vi "NACA_0015_Pressure_with_profile.vi"(3 "Mode":T5, 5 "Traverse line In":T1 {"Row Duration (mins)" format="%#.1f"; "Row No" min=0; "Trace Gas Concentration (%)" min=0.0 format="%#.2f"; "Emission Rate (l/min)" format="%#.2f"; "Tunnel Speed" format="%#.2f"; "Start X" format="%#.2f"; "Start Y" format="%#.2f"; "Start Z" format="%#.2f"; "End X" format="%#.2f"; "End Y" format="%#.2f"; "End Z" format="%#.2f"; "Averaging time (min)" min=0.0 format="%#.2f"}) -> (0 "Error Message":string, 1 "Status":T4, 2 "Traverse line Out":T1 {"Row Duration (mins)" format="%#.1f"; "Row No" min=0; "Trace Gas Concentration (%)" min=0.0 format="%#.2f"; "Emission Rate (l/min)" format="%#.2f"; "Tunnel Speed" format="%#.2f"; "Start X" format="%#.2f"; "Start Y" format="%#.2f"; "Start Z" format="%#.2f"; "End X" format="%#.2f"; "End Y" format="%#.2f"; "End Z" format="%#.2f"; "Averaging time (min)" min=0.0 format="%#.2f"})   [LabVIEW 2011]
uses:
  Gen Trav/Traverse_cluster.ctl
  Gen Trav/Spacing.ctl
  Controls/Multi_run_mode.ctl
  Controls/User_Specific_mode.ctl
  Gen Trav/Multi_Run_Status.ctl
  Gen Trav/Trav_mode.ctl
  Controls/Save_Data.ctl
  Controls/Setup.ctl
  <vilib>/Analysis/1siggen.llb/Ramp Pattern by Delta.vi
  <vilib>/Analysis/1siggen.llb/Ramp Pattern by Samples.vi
  Globals/Extra_Commands_Global.vi
  Globals/Meas_global.vi
  <vilib>/Analysis/NI_AALBase.lvlib
panel:
  out "Z":dbl
  out "Profile Points":cluster{dbl[], dbl[]}[](graph)
  out "Wake Profile":cluster{dbl[], dbl[]}(graph)
  in  "stop":bool
  out "Pressure":cluster{dbl[], dbl[]}(graph)
  out "Measurement No":i32
  # "X           Y            Z"
  # "Start"
  # "End"
  # "X           Y            Z"
  # "Start"
  # "End"
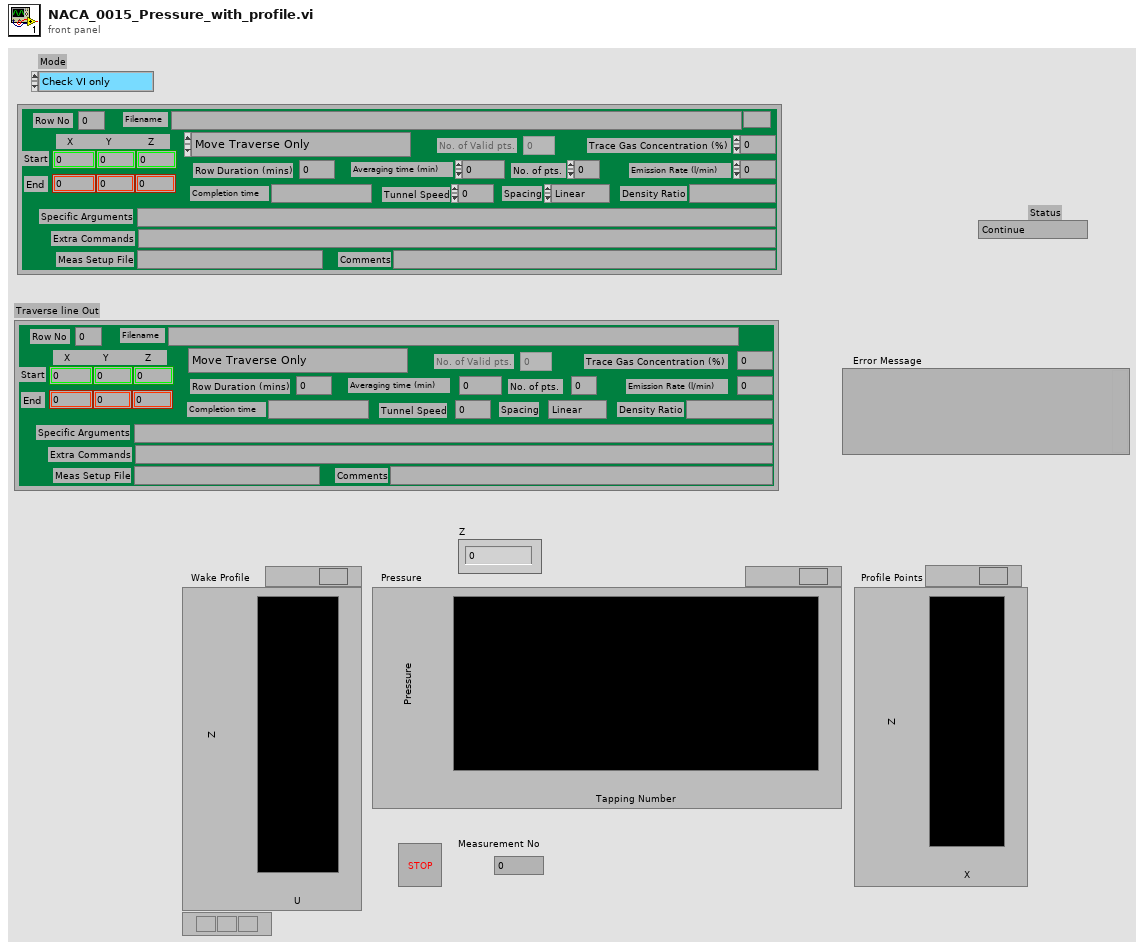
[diagram p1: front panel]
types:
  T1 = typedef "Traverse_cluster.ctl" = cluster{"Start X":dbl, "Start Y":dbl, "Start Z":dbl, "End X":dbl, "End Y":dbl, "End Z":dbl, "No. of pts.":i32, "Spacing":T2, "Filename":path, "Tunnel Speed":dbl, "Averaging time (min)":dbl, "Extra Commands":string, "Specific Arguments":string, "Emission Rate (l/min)":dbl, "Trace Gas Concentration (%)":dbl, "Density Ratio":string, "Comments":string, "Row No":i32, "Row Type Selector":T3, "Completion time":string, "Row Duration (mins)":dbl, "No. of Valid pts.":i32, "Meas Setup File":string}
  T2 = typedef "Spacing.ctl" = enum16{"Linear", "Log", "Gauss", "Specified", "N/A"}
  T3 = typedef "Multi_run_mode.ctl" = enum16{"Move Traverse Only", "Set Tunnel Speed Only", "Set Source Only", "Set Measurement Conditions", "Single Measurement", "Vertical Profile", "Lateral Profile", "Longitudinal Profile", "Explore Volume", "Multi-Axis Profile", "Auto Calibrate", "Meas Fast FID Bkgnd", "Check Beam Power", "Scanning Valve Measurement", "Run VI Named:", "Set ADAM Ch", "Wait (minutes)", "Send Message", "Synchronize With:", "Fall Back to this Row", "Turn Off Row Repeating", "Blank Row", "Traverse 3D Volume"}
  T4 = typedef "Multi_Run_Status.ctl" = enum16{"Continue", "Jump to Next Point", "Jump to Next Row", "Jump To Fall Back", "Terminate Run"}
  T5 = typedef "User_Specific_mode.ctl" = enum16{"Check VI only", "Run VI"}
  T6 = typedef "Trav_mode.ctl" = enum16{"Move traverse", "Read traverse position", "Teach Position"}
  T7 = typedef "Save_Data.ctl" = enum16{"Save No Data", "Save Data"}
  T8 = typedef "Setup.ctl" = enum16{"Run Program", "Show Setup", "Save Current Setup", "Setup Front Panel"}
  T9 = typedef "Status_Cluster.ctl" = cluster{"Status":T4, "Error Type":string, "Error Description":string}
  T10 = typedef "Analysis_info_cluster.ctl" = cluster{"Colour":u32, "Inst type":T11, "Inst name":string, "Symbol":string, "Code name":string, "Extra Info":string, "Inst Array":T12, "Extra Titles":string[], "Extra Values":string[], "U":dbl, "u^2":dbl, "u^3":dbl, "u^4":dbl, "Skew_u":dbl, "Kurt_u":dbl, "Sd Error in Mean":dbl, "% u'/U":dbl, "X":dbl, "Y":dbl, "Z":dbl, "Timescale integral to 25%":dbl, "Sd Error in Variance":dbl, "Calib File":path, "Calib Constants":dbl[], "Output Position":bool, "Full Stats":bool, "Av Sampling Rate":dbl, "Av No of Samples":dbl, "Total Meas Time (s)":dbl, "ADAM Ch Name":string}
  T11 = typedef "Inst_type.ctl" = enum16{"Propeller anemometer", "Raw voltage", "Pressure Transducer", "Pitot-static tube", "Preston tube", "Hot wire", "Cross wire 1", "Cross wire 2", "Generic Linear", "Generic Polynomial", "Generic BackPoly", "Fast FID", "Thermocouple", "Cold wire", "Pulsed Wire", "LDA Vel", "LDA Tran time", "LDA Arr time"}
  T12 = typedef "Instrument_Array.ctl" = enum16{"PWA", "LDA", "Analogue"}
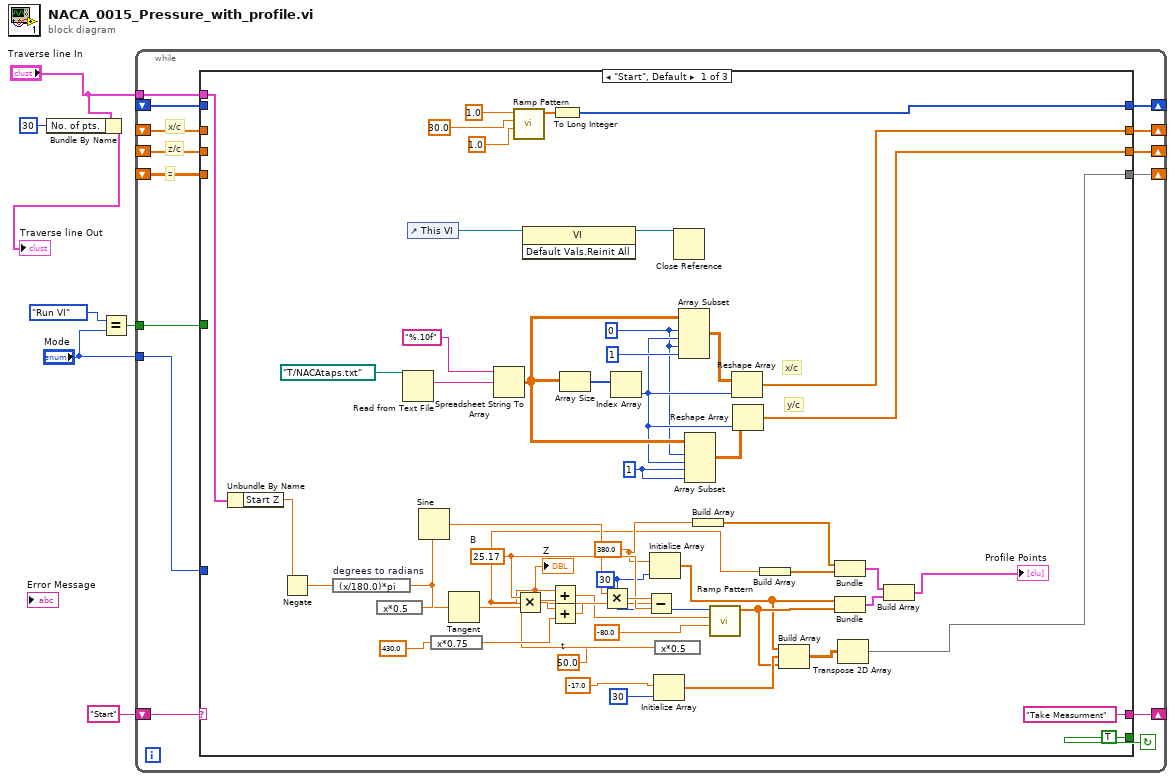
[diagram p0: block diagram]
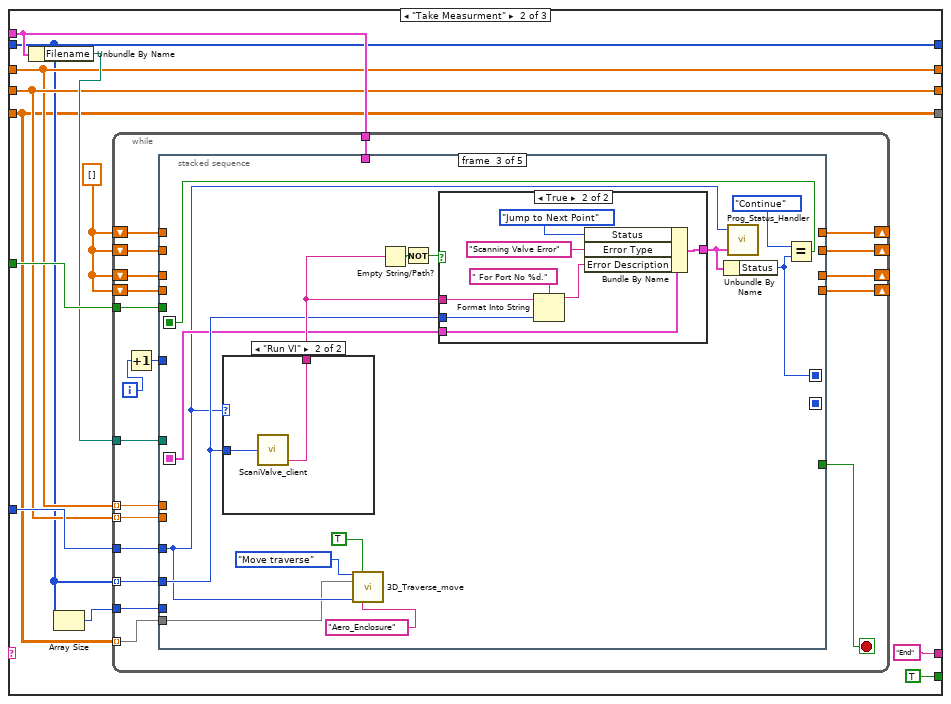
[diagram p2: hidden frame]
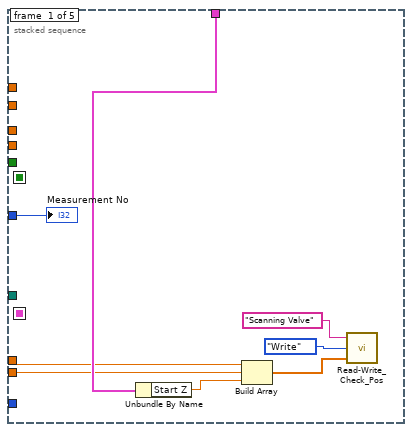
[diagram p3: hidden frame]
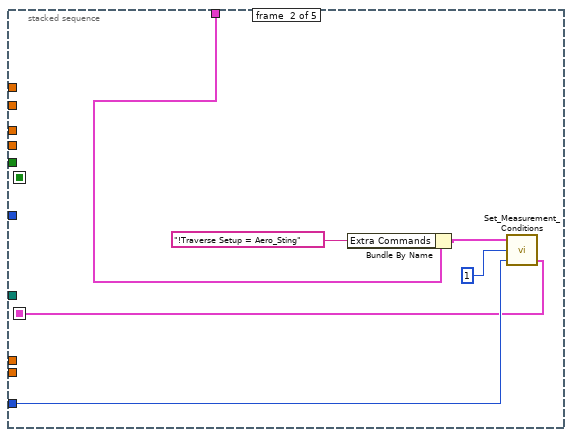
[diagram p4: hidden frame]
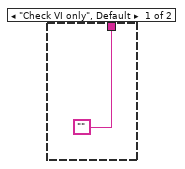
[diagram p5: hidden frame]
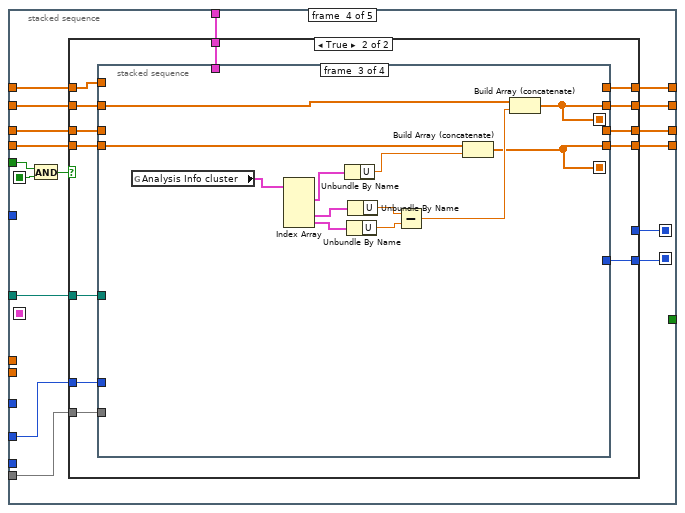
[diagram p7: hidden frame]
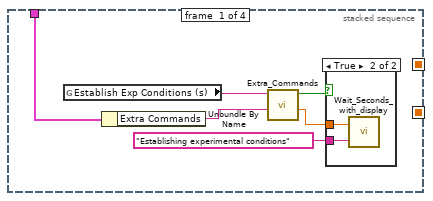
[diagram p9: hidden frame]
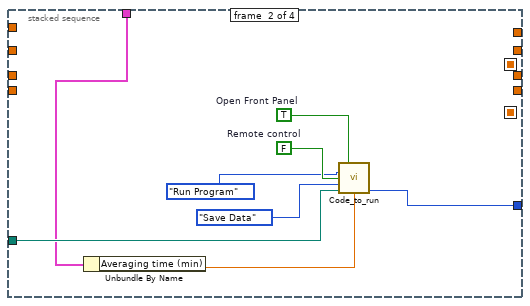
[diagram p11: hidden frame]
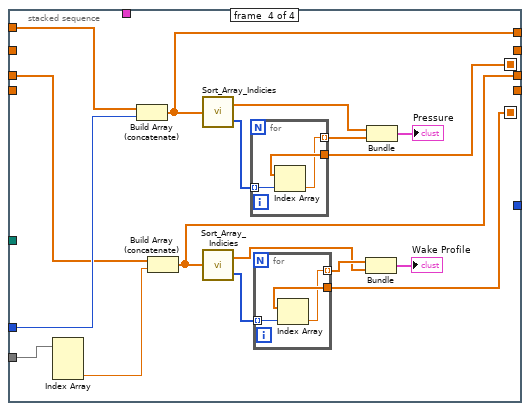
[diagram p12: hidden frame]
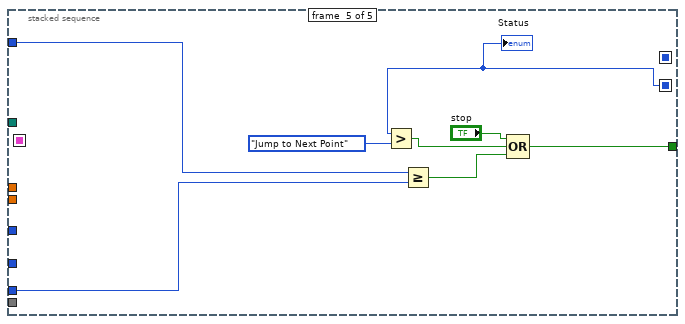
[diagram p13: hidden frame]
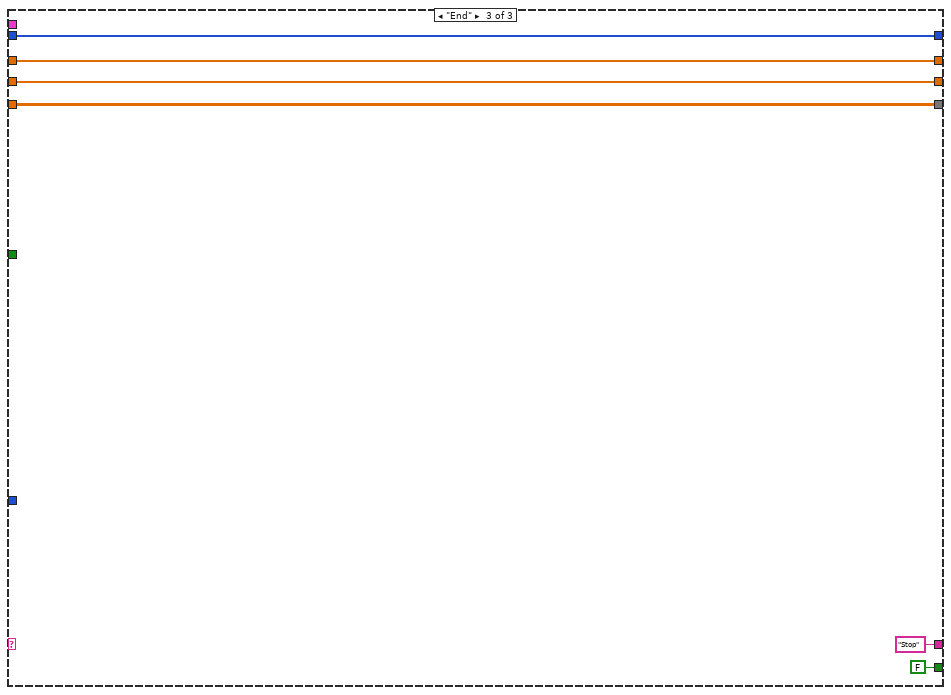
[diagram p14: hidden frame]
diagram:
  n1 = Bundle By Name(cluster="Traverse line In", "No. of pts."=30) -> (→"Traverse line Out":T1)
  n2 = Equal?(x=User_Specific_mode."Run VI" ("Mode"), y="Mode") -> (x = y?=w4:bool)
  n3 = while {
    tunnel: "Traverse line In" -> [w20]
    shift-right: [w19] -> _
    shift-left: "Start" -> [w18]
    tunnel: "Mode" -> [w17]
    tunnel: w4 -> [w16]
    shift-right: [w15] -> _
    shift-left: _ -> [w14]
    shift-right: [w13] -> _
    shift-left: _ -> [w11]
    shift-right: [w12] -> _
    shift-left: _ -> [w10]
    shift-right: [w9] -> _
    shift-left: _ -> [w8]
    stop <- w21 continue-if-true
    # "z"
    # "z/c"
    # "x/c"
    n4 = case shown="\"Start\", Default" w18 {
      tunnel: [TRUE TRUE FALSE] -> w21
      tunnel: w20 -> [w53 w84 _]
      tunnel: ["Take Measurment" "End" "Stop"] -> w19
      tunnel: w17 -> [_ w82 _]
      tunnel: w16 -> [_ w85 _]
      tunnel: [w71 w79 w245] -> w15
      tunnel: w14 -> [_ w79 w245]
      tunnel: [w57 w80 w244] -> w13
      tunnel: [w56 w81 w243] -> w12
      tunnel: w11 -> [_ w80 w244]
      tunnel: w10 -> [_ w81 w243]
      tunnel: [w22 w77 w242] -> w9
      tunnel: w8 -> [_ w77 w242]
      frame "Start", Default {
        w37 = 380.0 ("X")
        w41 = 30 ("samples")
        w33 = 50.0  # t
        w42 = 25.17  # B
        w58 = 1 ("index")
        w59 = 0 ("index")
        # "y/c"
        # "x/c"
        n5 = Unbundle By Name(w53) -> ("Start Z"=w24:dbl)
        n6 = Negate(x=w24) -> (-x=w34:dbl)
        n7 = expression code="(x/180.0)*pi" "degrees to radians"(w34) -> (w52:dbl)
        n8 = expression code="x*0.5"(w52) -> (w51:dbl)
        n9 = Read from Text File(file (use dialog)=path "T:/NACAtaps.txt") -> (text=w67:string)  [unwired: 3 in, 3 out]
        n10 = control-ref of="This VI"() -> (w55:refnum<vi>)
        n11 = Sine(x=w52) -> (sin(x)=w45:dbl)
        n12 = expression code="x*0.75"(430.0) -> (w47:dbl)
        n13 = Tangent(1:w51) -> (0:w50:dbl)
        n14 = Spreadsheet String To Array(format string="%.10f", spreadsheet string=w67) -> (array=w63:dbl[][])  [unwired: 2 in]
        n15 = call-poly <vilib>:"Ramp Pattern.vi"("start"=1.0, "end"=30.0, "delta"=1.0) -> ("Ramp Pattern"=w75:dbl[])  [unwired: 6 in, 2 out]
        n16 = Multiply(x=w42, y=w50) -> (x*y=w49:dbl)
        n17 = invoke class="VI" method="Default Vals.Reinit All"(reference=w55) -> (reference out=w54:refnum<vi>)  [unwired: 2 in, 2 out]
        n18 = Add(x=w49, y=w47) -> (x+y=w46:dbl)
        n19 = To Long Integer(number=w75) -> (32bit integer=w71:i32[])
        n20 = Array Size(array=w63) -> (size(s)=w65:i32[])
        n21 = Multiply(x=w45, y=w46) -> (x*y=w44:dbl)
        n22 = Index Array(array=w65) -> (element=w60:i32)  [unwired: 1 in]
        n23 = Subtract(x=w44, y=w42) -> (x-y=w32:dbl)
        "Z" <- w32
        n24 = Initialize Array(w37, w41) -> (w26:dbl[])
        n25 = Initialize Array(-17.0 ("Y"), 30 ("dimension size")) -> (w28:dbl[])
        n26 = expression code="x*0.5"(w33) -> (w43:dbl)
        n27 = Add(x=w32, y=w43) -> (x+y=w35:dbl)
        n28 = Close Reference(reference=w54) -> ()  [unwired: 1 in, 1 out]
        n29 = Array Subset(array=w63, index (row)=w59, length (row)=w60, index (col)=w59, length (col)=1 ("length")) -> (w62:dbl[][])
        n30 = Array Subset(array=w63, index (row)=w59, length (row)=w60, index (col)=w58, length (col)=w58) -> (w61:dbl[][])
        n31 = Build Array(w37) -> (w38:dbl[])
        n32 = call-poly <vilib>:"Ramp Pattern.vi"("start"=-80.0, "end"=w35, "samples"=w41) -> ("Ramp Pattern"=w27:dbl[])  [unwired: 7 in, 1 out]
        n33 = Reshape Array(w62, w60) -> (w57:dbl[])
        n34 = Reshape Array(w61, w60) -> (w56:dbl[])
        n35 = Build Array(w32) -> (w36:dbl[])
        n36 = Build Array(w26, w28, w27) -> (w25:dbl[][])
        n37 = Bundle(w38, w36) -> (w40:cluster{dbl[], dbl[]})  [unwired: 1 in]
        n38 = Bundle(w26, "Ramp Pattern"=w27) -> (w39:cluster{dbl[], "Ramp Pattern":dbl[]})  [unwired: 1 in]
        n39 = Transpose 2D Array(2D array=w25) -> (transposed array=w22:dbl[][])
        n40 = Build Array(w40, w39) -> (→"Profile Points":cluster{dbl[], "Ramp Pattern":dbl[]}[])
      }
      frame "Take Measurment" {
        w76 = dbl[] []
        n41 = Unbundle By Name(w84) -> ("Filename"=w83:path)
        n42 = Array Size(array=w79) -> (size(s)=w78:i32)
        n43 = while {
          tunnel: w82 -> [w102]
          tunnel: w85 -> [w99]
          tunnel: w83 -> [w107]
          shift-right: [w105] -> _
          shift-left: w76 -> [w106]
          shift-right: [w103] -> _
          shift-left: w76 -> [w104]
          tunnel: w84 -> [w101]
          tunnel: w79 -> [w96] mode=indexing
          tunnel: w80 -> [w95] mode=indexing
          tunnel: w81 -> [w94] mode=indexing
          tunnel: w78 -> [w93]
          tunnel: w77 -> [w92] mode=indexing
          shift-right: [w91] -> _
          shift-left: w76 -> [w90]
          shift-right: [w88] -> _
          shift-left: w76 -> [w89]
          i -> [w98]
          stop <- w100 stop-if-true
          n44 = Increment(x=w98) -> (x+1=w97:i32)
          n45 = stacked-sequence {
            seq-local: [_ _ w130 _ _] -> [_ _ _ w156 _]
            seq-local: [_ _ w129 _ _] -> [_ _ _ w157 _]
            seq-local: [_ _ _ w158 _] -> [_ _ _ _ w235]
            seq-local: [_ w116 _ _ _] -> [_ _ w127 _ _]
            tunnel: w107 -> [_ _ _ w164 _]
            tunnel: w106 -> [_ _ _ w163 _]
            tunnel: [_ _ _ w162 _] -> w105
            tunnel: w104 -> [_ _ _ w161 _]
            tunnel: [_ _ _ w160 _] -> w103
            tunnel: w102 -> [_ w117 w125 _ _]
            tunnel: w101 -> [w114 w118 _ w159 _]
            tunnel: w97 -> [w115 _ _ _ w238]
            tunnel: [_ _ _ _ w236] -> w100
            tunnel: w99 -> [_ _ _ w155 _]
            tunnel: w96 -> [_ _ w128 w153 _]
            tunnel: w95 -> [w113 _ _ _ _]
            tunnel: w94 -> [w112 _ _ _ _]
            tunnel: w93 -> [_ _ _ _ w234]
            tunnel: w92 -> [_ _ w122 w152 _]
            tunnel: [_ _ _ w151 _] -> w91
            tunnel: w90 -> [_ _ _ w150 _]
            tunnel: w89 -> [_ _ _ w149 _]
            tunnel: [_ _ _ w148 _] -> w88
            frame #0 {
              n46 = Unbundle By Name(w114) -> ("Start Z"=w111:dbl)
              n47 = Build Array(w113, w112, w111) -> (w110:dbl[])
              n48 = call "Read-Write_Check_Pos.vi"("Position input"=w110, "Mode"=enum16{"Read", "Write"}."Write", "Traverse Name"="Scanning Valve") -> ()  [unwired: 1 out]
              "Measurement No" <- w115
            }
            frame #1 {
              n49 = Bundle By Name(cluster=w118, "Extra Commands"="!Traverse Setup = Aero_Sting") -> (w121:T1)
              n50 = call "Set_Measurement_Conditions.vi"("Simulate/Run"=w117, "Currently on Point"=1, "Traverse line"=w121) -> ("Status Cluster"=w116:T9)  [unwired: 2 in]
            }
            frame #2 {
              n51 = case shown="\"Run VI\"" w125 {
                tunnel: w128 -> [_ w138]
                tunnel: ["" w137] -> w133
                frame "Check VI only", Default {
                }
                frame "Run VI" {
                  n52 = call "ScaniValve_client.vi"("Port Number"=w138) -> ("Error String"=w137:string)  [unwired: 2 out]
                }
              }
              n53 = call "3D_Traverse_move.vi"("Mode"=Trav_mode."Move traverse", "Route Checking?"=TRUE, "Position"=w122, "Simulate/Run"=w125, "Traverse name"="Aero_Enclosure" ("Traverse Name")) -> ()  [unwired: 8 in, 3 out]
              n54 = Empty String/Path?(string/path=w133) -> (empty?=w135:bool)
              n55 = Not(x=w135) -> (.not. x?=w134:bool)
              n56 = case shown="True" w134 {
                tunnel: w127 -> [w139 w147]
                tunnel: [w139 w144] -> w131
                tunnel: w133 -> [_ w141]
                tunnel: w128 -> [_ w140]
                frame False {
                }
                frame True {
                  n57 = Format Into String(format string=" For Port No %d." ("Format String"), initial string=w141, w140) -> (resulting string=w142:string)  [unwired: 1 in, 1 out]
                  n58 = Bundle By Name(cluster=w147, "Status"=Multi_Run_Status."Jump to Next Point", "Error Type"="Scanning Valve Error" ("t"), "Error Description"=w142) -> (w144:T9)
                }
              }
              n59 = Unbundle By Name(w131) -> ("Status"=w129:T4)
              n60 = call "Prog_Status_Handler.vi"("Status Cluster"=w131, "Simulate/Run"=w125) -> ()  [unwired: 2 out]
              n61 = Equal?(x=Multi_Run_Status."Continue" ("Status"), y=w129) -> (x = y?=w130:bool)
            }
            frame #3 {
              n62 = And(x=w155, y=w156) -> (x .and. y?=w154:bool)
              n63 = case shown="True" w154 {
                tunnel: [w167 w182] -> w158
                tunnel: w164 -> [_ w181]
                tunnel: w163 -> [w169 w180]
                tunnel: [w169 w179] -> w162
                tunnel: w161 -> [w168 w178]
                tunnel: [w168 w177] -> w160
                tunnel: w159 -> [_ w176]
                tunnel: w153 -> [_ w175]
                tunnel: w157 -> [w167 _]
                tunnel: w152 -> [_ w174]
                tunnel: [w165 w173] -> w151
                tunnel: w150 -> [w165 w172]
                tunnel: w149 -> [w166 w171]
                tunnel: [w166 w170] -> w148
                frame False {
                }
                frame True {
                  n64 = stacked-sequence {
                    seq-local: [_ _ w209 _] -> [_ _ _ w222]
                    seq-local: [_ _ w200 _] -> [_ _ _ w217]
                    tunnel: [_ w193 _ _] -> w182
                    tunnel: w181 -> [_ w192 _ _]
                    tunnel: w180 -> [_ _ w210 _]
                    tunnel: [_ _ w209 _] -> w179
                    tunnel: w178 -> [_ _ _ w227]
                    tunnel: [_ _ _ w225] -> w177
                    tunnel: w176 -> [w188 w191 _ _]
                    tunnel: w175 -> [_ _ _ w220]
                    tunnel: w174 -> [_ _ _ w219]
                    tunnel: [_ _ w200 _] -> w173
                    tunnel: w172 -> [_ _ w199 _]
                    tunnel: w171 -> [_ _ _ w212]
                    tunnel: [_ _ _ w211] -> w170
                    frame #0 {
                      n65 = global read "Extra_Commands_Global.vi" "Establish Exp Conditions (s)"() -> (w185:string)
                      n66 = Unbundle By Name(w188) -> ("Extra Commands"=w187:string)
                      n67 = call "Extra_Commands.vi"("String to Search"=w187, "Command"=w185) -> ("Numeric Value"=w186:dbl, "Command Found"=w184:bool)  [unwired: 2 in, 2 out]
                      n68 = case shown="True" w184 {
                        tunnel: w186 -> [_ w190]
                        tunnel: "Establishing experimental conditions" ("Message") -> [_ w189]
                        frame False {
                        }
                        frame True {
                          n69 = call "Wait_Seconds_with_display.vi"("Message"=w189, "Seconds to wait"=w190) -> ()  [unwired: 1 in, 1 out]
                        }
                      }
                    }
                    frame #1 {
                      w196 = TRUE  # Open Front Panel
                      w198 = FALSE  # Remote control
                      n70 = Unbundle By Name(w191) -> ("Averaging time (min)"=w197:dbl)
                      n71 = call "Code_to_run.vi"("Open Front Panel"=w196, "setup"=Setup."Run Program", "Remote control"=w198, "File"=Save_Data."Save Data", "Results Filename"=w192, "Averaging time (min)"=w197) -> ("Status"=w193:T4)  [unwired: 5 in, 4 out]
                    }
                    frame #2 {
                      n72 = global read "Meas_global.vi" "Analysis Info cluster"() -> (w208:T10[])
                      n73 = Index Array(array=w208) -> (element #1=w202:T10, element #3=w203:T10, element #4=w204:T10)  [unwired: 4 in, 1 out]
                      n74 = Unbundle By Name(w202) -> ("U"=w201:dbl)
                      n75 = Unbundle By Name(w204) -> ("U"=w205:dbl)
                      n76 = Unbundle By Name(w203) -> ("U"=w206:dbl)
                      n77 = Subtract(x=w206, y=w205) -> (x-y=w207:dbl)
                      n78 = Build Array (concatenate)(w199, w201) -> (w200:dbl[])
                      n79 = Build Array (concatenate)(w210, w207) -> (w209:dbl[])
                    }
                    frame #3 {
                      n80 = Index Array(array=w219) -> (element #3=w213:dbl)  [unwired: 3 in, 2 out]
                      n81 = Build Array (concatenate)(w227, w220) -> (w225:dbl[])
                      n82 = Build Array (concatenate)(w212, w213) -> (w211:dbl[])
                      n83 = call "Sort_Array_Indicies.vi"("unsorted array"=w225) -> ("sorted array"=w224:dbl[], "Sort Index"=w223:i32[])
                      n84 = call "Sort_Array_Indicies.vi"("unsorted array"=w211) -> ("sorted array"=w214:dbl[], "Sort Index"=w218:i32[])
                      n85 = for {
                        tunnel: w223 -> [w233] mode=indexing
                        tunnel: w222 -> [w232]
                        tunnel: [w231] -> w221 mode=indexing
                        n86 = Index Array(array=w232, index=w233) -> (element=w231:dbl)
                      }
                      n87 = for {
                        tunnel: w218 -> [w230] mode=indexing
                        tunnel: w217 -> [w229]
                        tunnel: [w228] -> w215 mode=indexing
                        n88 = Index Array(array=w229, index=w230) -> (element=w228:dbl)
                      }
                      n89 = Bundle(w215, "sorted array"=w214) -> (→"Wake Profile":cluster{dbl[], "sorted array":dbl[]})  [unwired: 1 out]
                      n90 = Bundle("sorted array"=w224, w221) -> (→"Pressure":cluster{"sorted array":dbl[], dbl[]})  [unwired: 1 out]
                    }
                  }
                }
              }
            }
            frame #4 {
              n91 = Greater?(x=w235, y=Multi_Run_Status."Jump to Next Point" ("Status")) -> (0:w240:bool)
              n92 = Greater Or Equal?(x=w238, y=w234) -> (x >= y?=w239:bool)
              n93 = Compound Arithmetic op=OR("stop", w240, w239) -> (w236:bool)
              "Status" <- w235
            }
          }
        }
      }
      frame "End" {
      }
    }
  }
